vi "DMAsOverflow.vi"() -> (2 "DMAsOverFlow":u16)   [LabVIEW 2013]
uses:
  vis5761/libs/common/GlobalReg.vi
  vis5761/libs/IRIO.lvlib
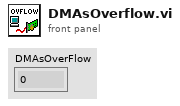
[diagram p1: front panel]
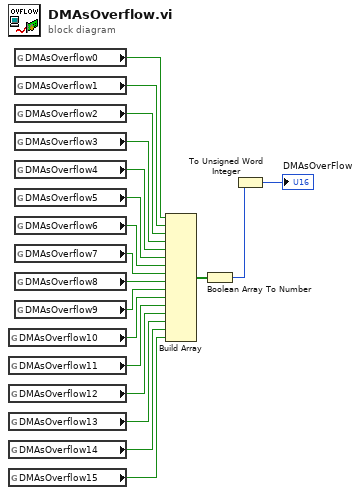
[diagram p0: block diagram]
diagram:
  n1 = global read "GlobalReg.vi" "DMAsOverflow10"() -> (w6:bool)
  n2 = global read "GlobalReg.vi" "DMAsOverflow11"() -> (w5:bool)
  n3 = global read "GlobalReg.vi" "DMAsOverflow12"() -> (w4:bool)
  n4 = global read "GlobalReg.vi" "DMAsOverflow13"() -> (w3:bool)
  n5 = global read "GlobalReg.vi" "DMAsOverflow14"() -> (w2:bool)
  n6 = global read "GlobalReg.vi" "DMAsOverflow15"() -> (w1:bool)
  n7 = global read "GlobalReg.vi" "DMAsOverflow0"() -> (w16:bool)
  n8 = global read "GlobalReg.vi" "DMAsOverflow1"() -> (w15:bool)
  n9 = global read "GlobalReg.vi" "DMAsOverflow2"() -> (w14:bool)
  n10 = global read "GlobalReg.vi" "DMAsOverflow3"() -> (w13:bool)
  n11 = global read "GlobalReg.vi" "DMAsOverflow4"() -> (w12:bool)
  n12 = global read "GlobalReg.vi" "DMAsOverflow5"() -> (w11:bool)
  n13 = global read "GlobalReg.vi" "DMAsOverflow6"() -> (w10:bool)
  n14 = global read "GlobalReg.vi" "DMAsOverflow7"() -> (w9:bool)
  n15 = global read "GlobalReg.vi" "DMAsOverflow8"() -> (w8:bool)
  n16 = global read "GlobalReg.vi" "DMAsOverflow9"() -> (w7:bool)
  n17 = Build Array(w16, w15, w14, w13, w12, w11, w10, w9, w8, w7, w6, w5, w4, w3, w2, w1) -> (w19:bool[])
  n18 = Boolean Array To Number(Boolean array=w19) -> (number=w18:u16)
  n19 = To Unsigned Word Integer(number=w18) -> (unsigned 16bit integer=→"DMAsOverFlow":u16)
